vi "Integrate.vi"(1 "Input Array Y":dbl[](array[numeric]), 2 "Input Array X":dbl[](array[numeric])) -> (0 "Output Array":dbl[](array[numeric]))   [LabVIEW 2016]
panel:
  out "Waveform Graph 3":dbl[](graph)
  out "Waveform Graph 2":dbl[](graph)
  out "Waveform Graph":dbl[](graph)
  out "x-y":dbl
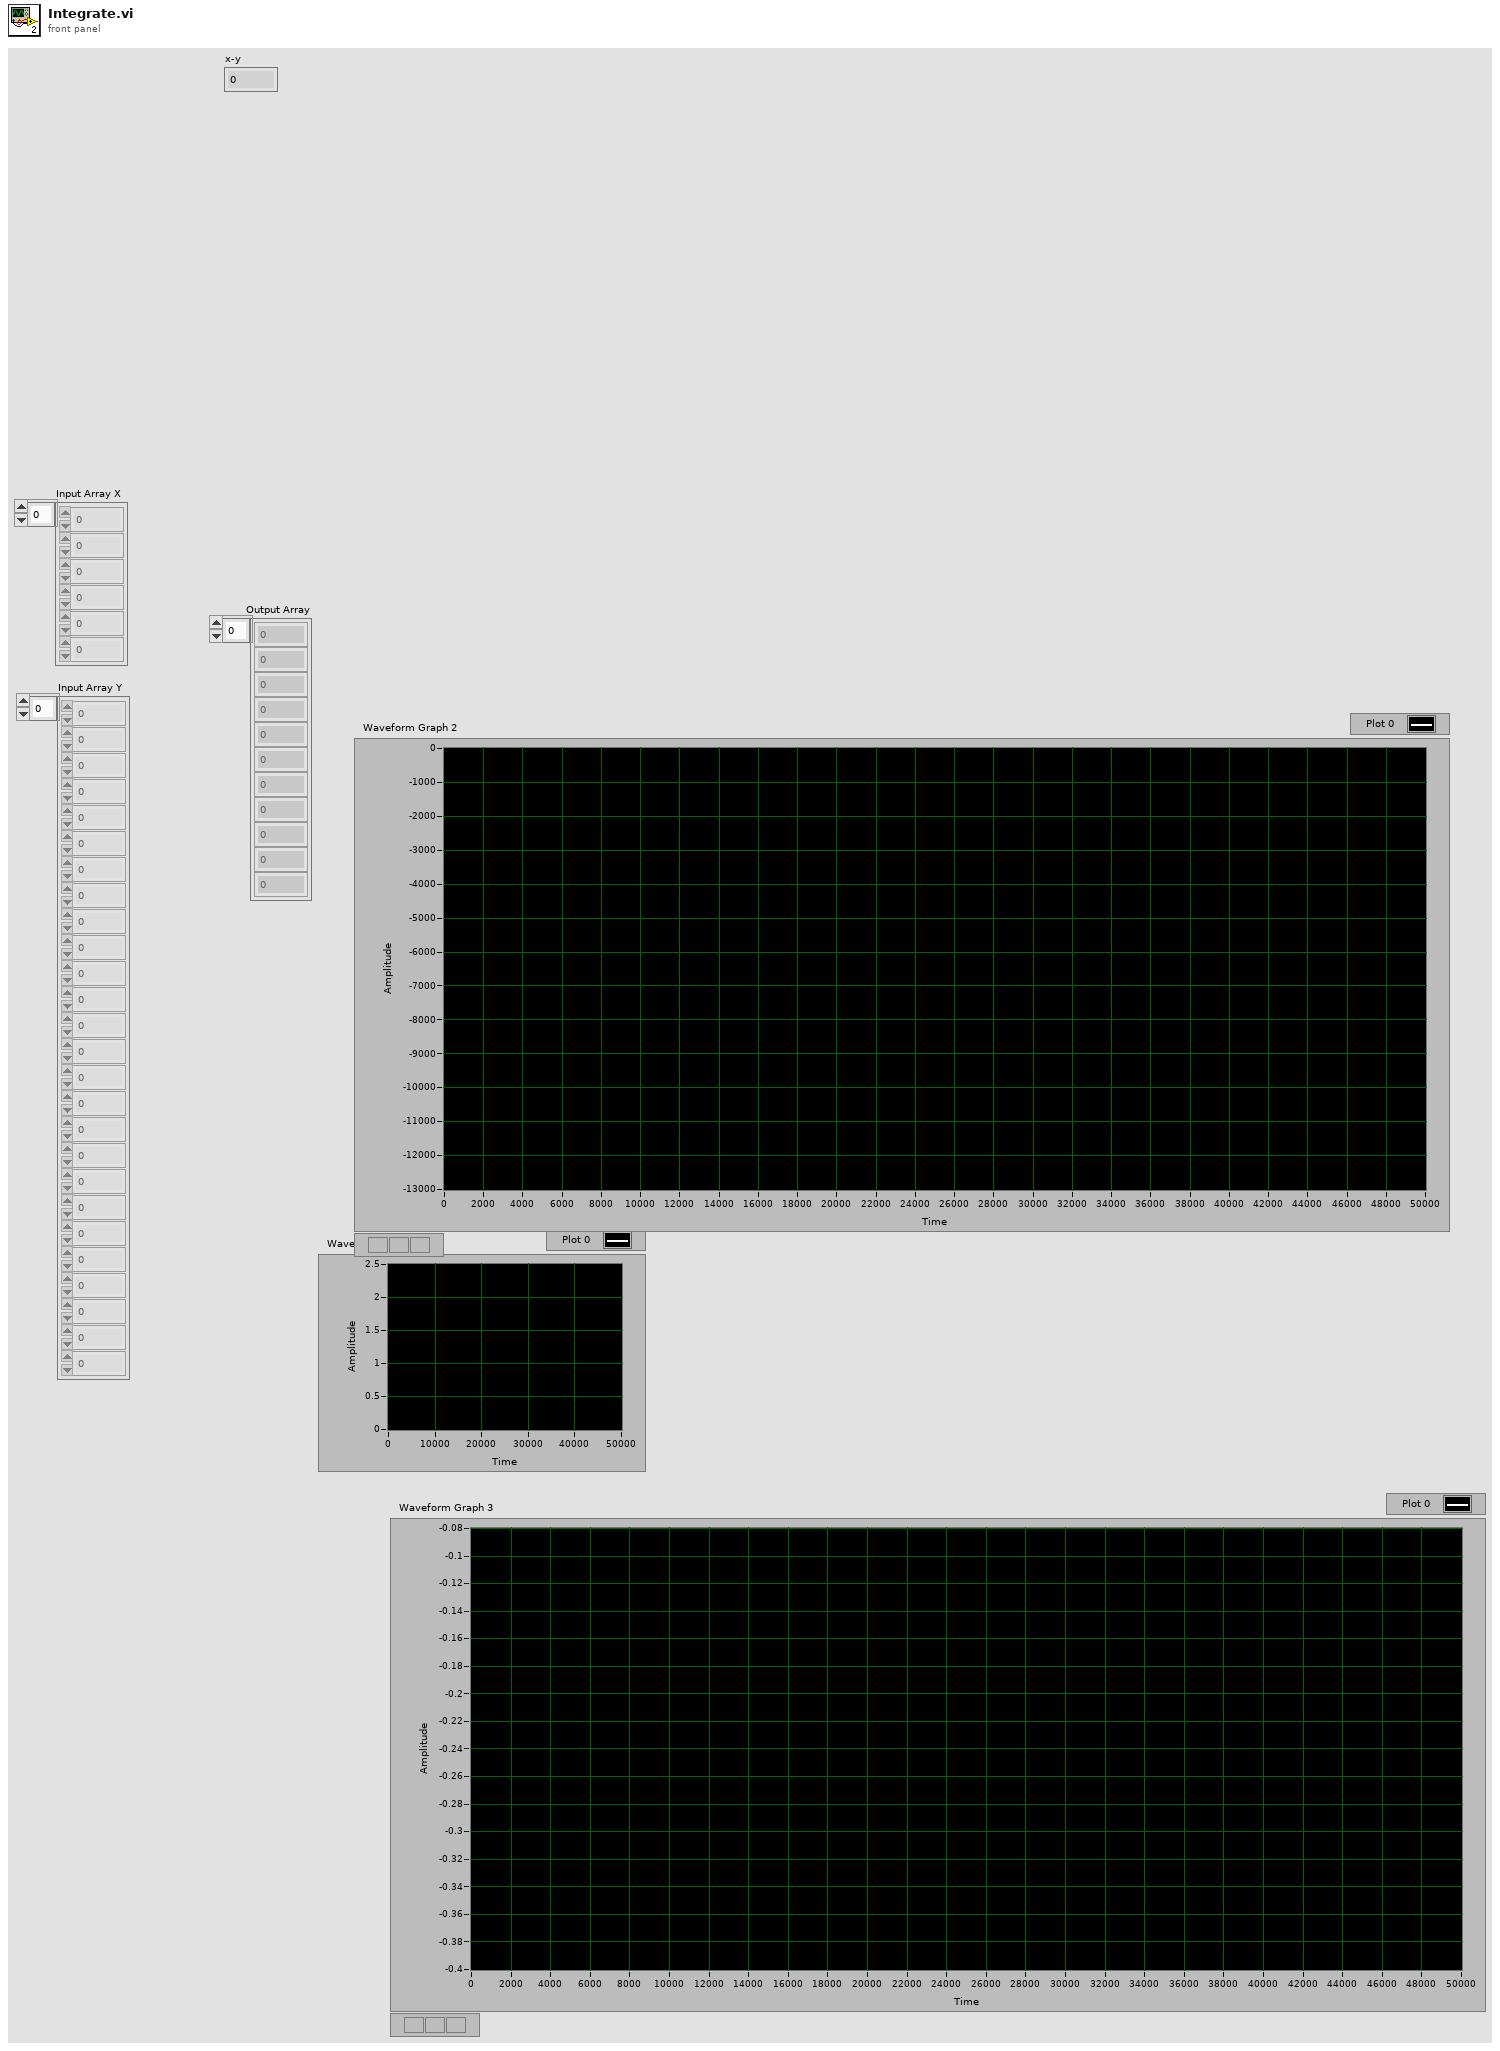
[diagram p1: front panel]
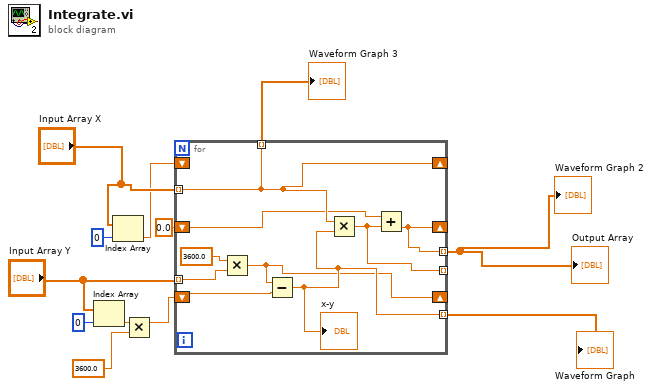
[diagram p0: block diagram]
diagram:
  n1 = Index Array(array="Input Array Y", index=0) -> (element=w8:dbl)
  n2 = Index Array(array="Input Array X", index=0) -> (element=w5:dbl)
  n3 = Multiply(x=w8, y=3600.0 ("x")) -> (x*y=w3:dbl)
  n4 = for {
    shift-right: [w14] -> _
    shift-left: w3 -> [w21]
    tunnel: "Input Array Y" -> [w20] mode=indexing
    tunnel: "Input Array X" -> [w18] mode=indexing
    shift-right: [w18] -> _
    shift-left: w5 -> [_]
    tunnel: [w17] -> w1 mode=indexing
    tunnel: [w19] -> w7 mode=indexing
    tunnel: [w18] -> w6 mode=indexing
    shift-right: [w17] -> _
    shift-left: 0.0 -> [w16]
    tunnel: [w15] -> _ mode=indexing
    n5 = Multiply(x=3600.0, y=w20) -> (x*y=w14:dbl)
    n6 = Subtract(x=w14, y=w21) -> (x-y=w19:dbl)
    "x-y" <- w19
    n7 = Multiply(x=w18, y=w19) -> (x*y=w15:dbl)
    n8 = Add(x=w16, y=w15) -> (x+y=w17:dbl)
  }
  "Output Array" <- w1
  "Waveform Graph" <- w7
  "Waveform Graph 2" <- w1
  "Waveform Graph 3" <- w6
